vi "image_grap.vi"() -> ()   [LabVIEW 2020]
uses:
  <vilib>/userdefined/High Color/IMAQdx.ctl
  <vilib>/vision/driver/NI_Vision_Acquisition_Software.lvlib
panel:
  out "Image":T1(plugin-control)
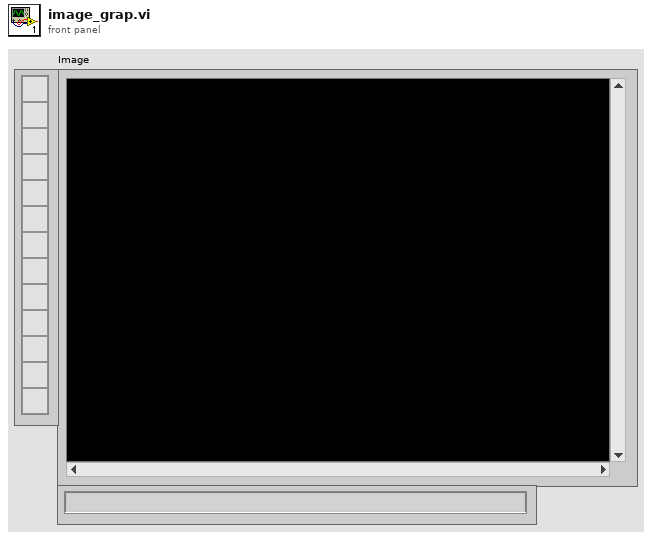
[diagram p1: front panel]
types:
  T1 = typedef "IMAQ Image.ctl" = refnum<image>
  T2 = typedef "IMAQdx.ctl" = refnum<k21>
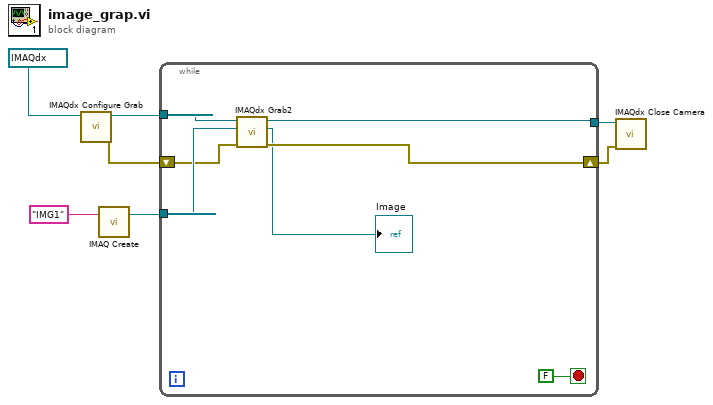
[diagram p0: block diagram]
diagram:
  n1 = call <vilib>:"IMAQdx Configure Grab.vi"("Session In"=T2 "cam0") -> ("error out"=w3:errorcluster, "Session Out"=w5:T2)  [unwired: 9 in]
  n2 = call "IMAQ Create"("Image Name"="IMG1") -> ("New Image"=w4:T1)  [unwired: 4 in, 1 out]
  n3 = while {
    tunnel: w5 -> [w14]
    tunnel: w4 -> [w13]
    shift-right: [w11] -> w2
    shift-left: w3 -> [w12]
    tunnel: [w9] -> w1
    stop <- FALSE stop-if-true
    n4 = call <vilib>:"IMAQdx Grab2.vi"("error in"=w12, "Image In"=w13, "Session In"=w14) -> ("error out"=w11:errorcluster, "Image Out"=→"Image":T1, "Session Out"=w9:T2)  [unwired: 5 in, 1 out]
  }
  n5 = call <vilib>:"IMAQdx Close Camera.vi"("error in"=w2, "Session In"=w1) -> ()  [unwired: 9 in, 1 out]
